vi "Spartan HTTP Startup.vi"(4 "error in (no error)":errorcluster) -> (0 "error out":errorcluster, 3 "Startup Message":string)   [LabVIEW 2011]
uses:
  Addons/internet/http/http0.llb/HTTP LVHTTP Global.vi
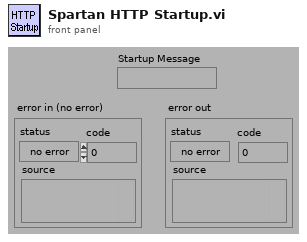
[diagram p1: front panel]
types:
  T1 = enum16{"get", "reserve", "free", "compact", "empty", "status"}
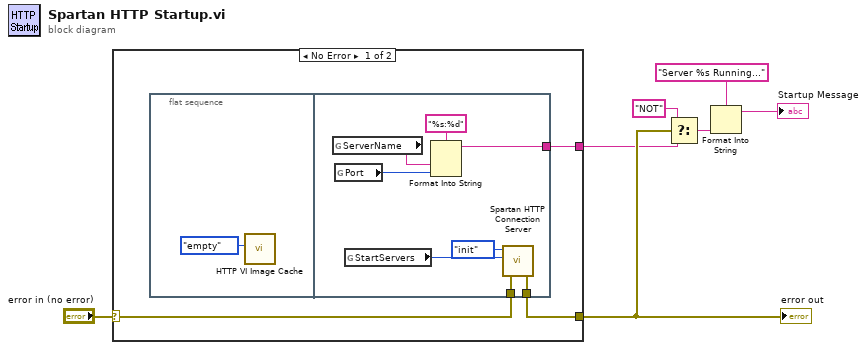
[diagram p0: block diagram]
diagram:
  n1 = case shown="No Error" "error in (no error)" {
    selector: "error in (no error)" -> [w10 w20]
    tunnel: [w9 w20] -> w4
    tunnel: [w8 _] -> w1
    frame No Error {
      n2 = flat-sequence {
        tunnel: [w16] -> w8
        tunnel: w10 -> [w15]
        tunnel: [w14] -> w9
        frame #0 {
          n3 = call "HTTP VI Image Cache.vi"("function (get)"=T1."empty") -> ()  [unwired: 3 in, 8 out]
        }
        frame #1 {
          n4 = global read "HTTP LVHTTP Global.vi" "ServerName"() -> (w18:string)
          n5 = global read "HTTP LVHTTP Global.vi" "Port"() -> (w17:u16)
          n6 = global read "HTTP LVHTTP Global.vi" "StartServers"() -> (w13:i32)
          n7 = Format Into String(format string="%s:%d", w18, w17) -> (resulting string=w16:string)  [unwired: 2 in, 1 out]
          n8 = call "Spartan HTTP Connection Server.vi"("error in (no error)"=w15, "Handlers to Init (4)"=w13, "function (init)"=enum16{"init", "finish"}."init") -> ("error out"=w14:errorcluster)  [unwired: 4 out]
        }
      }
    }
    frame Error {
    }
  }
  "error out" <- w4
  n9 = Select(t="NOT", s=w4, f=w1) -> (s? t:f=w2:string)
  n10 = Format Into String(format string="Server %s Running...", w2) -> (resulting string=→"Startup Message":string)  [unwired: 2 in, 1 out]
